vi "decrement N attempt.vi"(8 "error in (no error)":errorcluster, 11 "Master CR in":refnum<class "WebSocket Client CR.lvclass">) -> (0 "error out":errorcluster, 2 "=0":bool, 3 "Master CR out":refnum<class "WebSocket Client CR.lvclass">)   [LabVIEW 2021, in "WebSockets.lvlib" / "WebSocket Client CR.lvclass"]
uses:
  WebSocket Client CR.lvclass
  WebSocket Client CR.lvclass/WebSocket Client CR.ctl
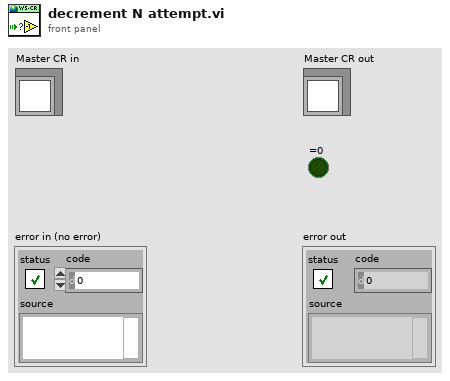
[diagram p1: front panel]
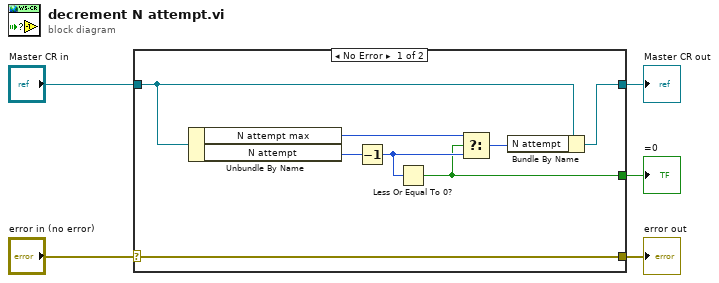
[diagram p0: block diagram]
diagram:
  n1 = case shown="No Error" "error in (no error)" {
    selector: "error in (no error)" -> [w13 w14]
    tunnel: [w13 w14] -> w4
    tunnel: [w12 w15] -> w2
    tunnel: "Master CR in" -> [w11 w15]
    tunnel: [w7 _] -> w1
    frame No Error {
      n2 = Unbundle By Name(w11) -> ("N attempt max"=w6:i32, "N attempt"=w10:i32)
      n3 = Decrement(x=w10) -> (x-1=w9:i32)
      n4 = Less Or Equal To 0?(x=w9) -> (x <= 0?=w7:bool)
      n5 = Select(t=w6, s=w7, f=w9) -> (s? t:f=w8:i32)
      n6 = Bundle By Name(cluster=w11, "N attempt"=w8) -> (w12:refnum<class "WebSocket Client CR.lvclass">)
    }
    frame Error {
    }
  }
  "error out" <- w4
  "Master CR out" <- w2
  "=0" <- w1
